vi "Page_Advanced_ReadShared.vi"(6 "ctl references":T1, 8 "error in (no error)":errorcluster, 11 "AB_Build in":refnum<class "AB_Build.lvclass">) -> (0 "error out":errorcluster, 3 "AB_Build out":refnum<class "AB_Build.lvclass">)   [LabVIEW 2020, in "AB_Build.lvclass"]
uses:
  <vilib>/AppBuilder/AB_Classes/Build/AB_Build.lvclass
  <resource>/Framework/Providers/Builds/AppBuilder/AB_UI_Page_Advanced_References.ctl
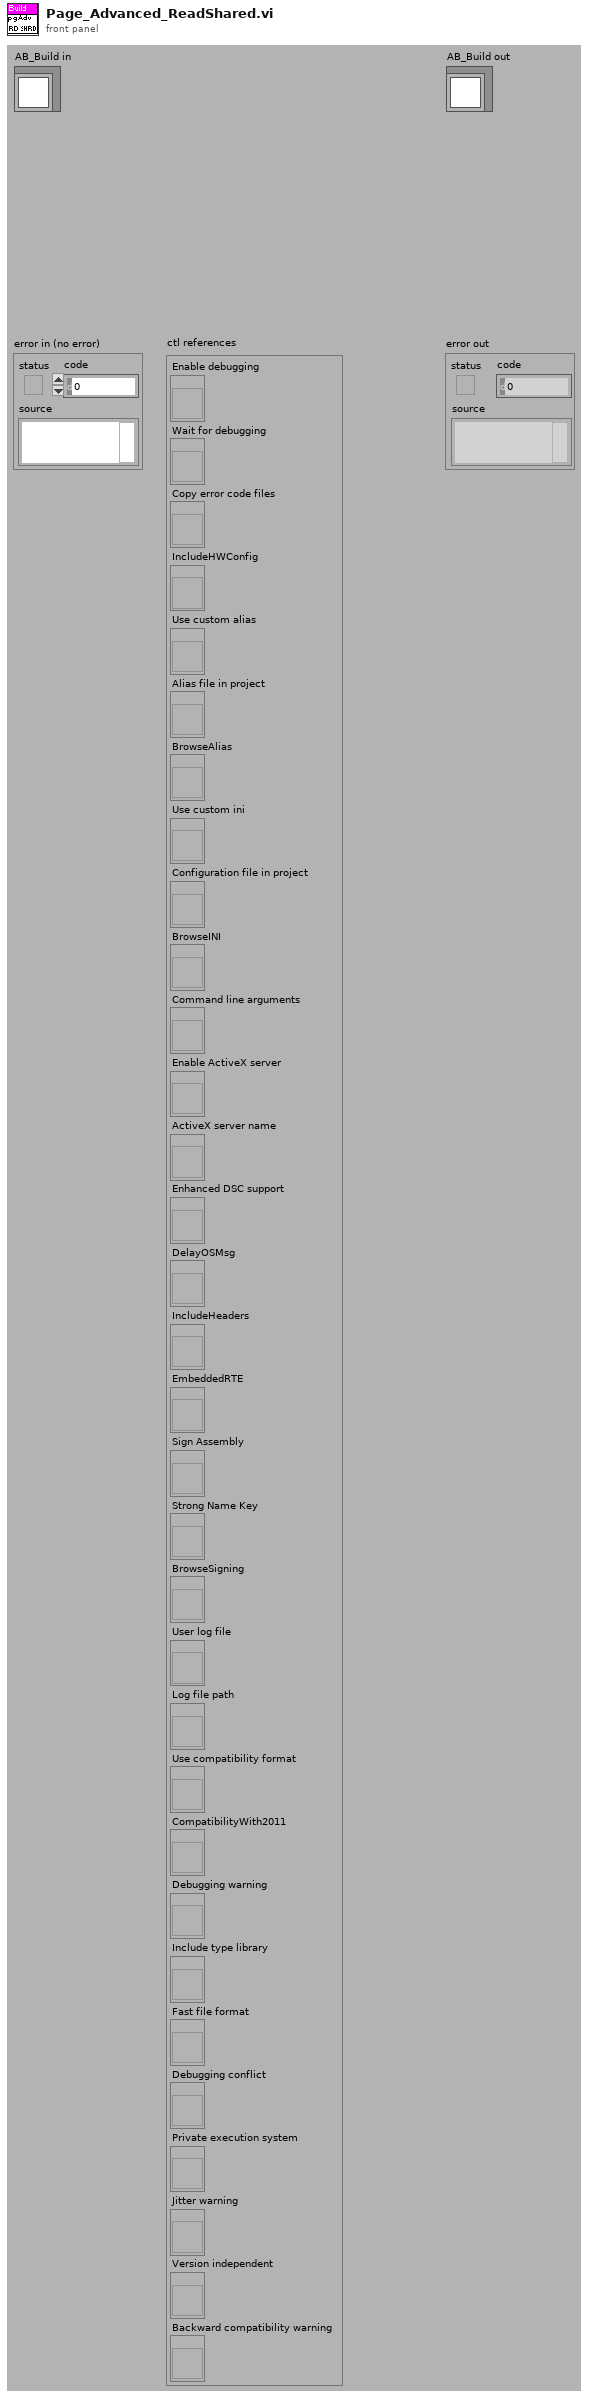
[diagram p1: front panel]
types:
  T1 = typedef "AB_UI_Page_Advanced_References.ctl" = cluster{"Enable debugging":refnum<vi>, "Wait for debugging":refnum<vi>, "Copy error code files":refnum<vi>, "IncludeHWConfig":refnum<vi>, "Use custom alias":refnum<vi>, "Alias file in project":refnum<vi>, "BrowseAlias":refnum<vi>, "Use custom ini":refnum<vi>, "Configuration file in project":refnum<vi>, "BrowseINI":refnum<vi>, "Command line arguments":refnum<vi>, "Enable ActiveX server":refnum<vi>, "ActiveX server name":refnum<vi>, "Enhanced DSC support":refnum<vi>, "DelayOSMsg":refnum<vi>, "IncludeHeaders":refnum<vi>, "EmbeddedRTE":refnum<vi>, "Sign Assembly":refnum<vi>, "Strong Name Key":refnum<vi>, "BrowseSigning":refnum<vi>, "User log file":refnum<vi>, "Log file path":refnum<vi>, "Use compatibility format":refnum<vi>, "CompatibilityWith2011":refnum<vi>, "Debugging warning":refnum<vi>, "Include type library":refnum<vi>, "Fast file format":refnum<vi>, "Debugging conflict":refnum<vi>, "Private execution system":refnum<vi>, "Jitter warning":refnum<vi>, "Version independent":refnum<vi>, "Backward compatibility warning":refnum<vi>}
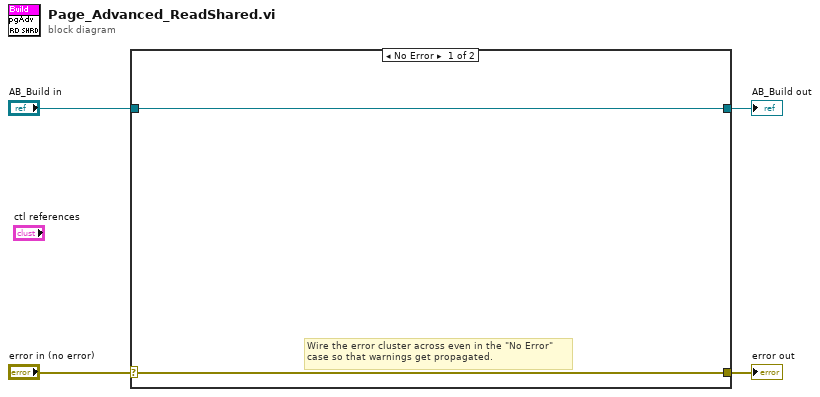
[diagram p0: block diagram]
diagram:
  n1 = case shown="No Error" "error in (no error)" {
    selector: "error in (no error)" -> [w5 w8]
    tunnel: [w5 w8] -> w3
    tunnel: [w6 w7] -> w1
    tunnel: "AB_Build in" -> [w6 w7]
    frame No Error {
      # "Wire the error cluster across even in the \"No Error\"\ncase so that warnings get propagated."
    }
    frame Error {
    }
  }
  "error out" <- w3
  "AB_Build out" <- w1
